vi "ChangeGrating.vi"(8 "error in (no error)":errorcluster, 10 "Grating":enum16{"Mirror", "1200 g/mm", "1800 g/mm"}(ring), 11 "HRS_Spectrometer in":refnum<class "HRS_Spectrometer.lvclass">) -> (0 "error out":errorcluster, 3 "HRS_Spectrometer out":refnum<class "HRS_Spectrometer.lvclass">)   [LabVIEW 2023, in "HRS_Spectrometer.lvlib" / "HRS_Spectrometer.lvclass"]
uses:
  HRS_Spectrometer.lvclass
  HRS_Spectrometer.lvclass/HRS_Spectrometer.ctl
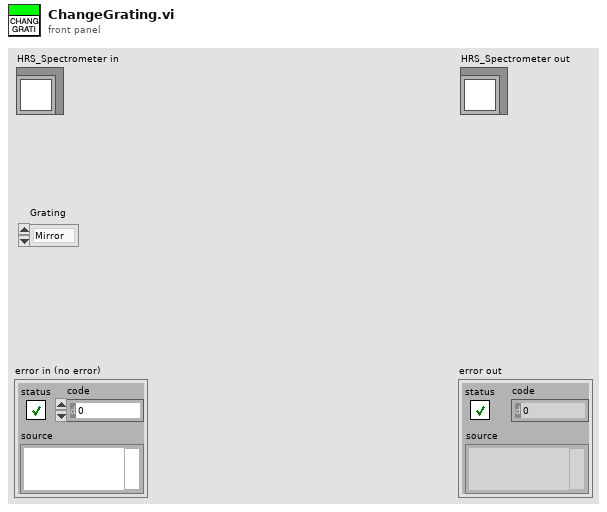
[diagram p1: front panel]
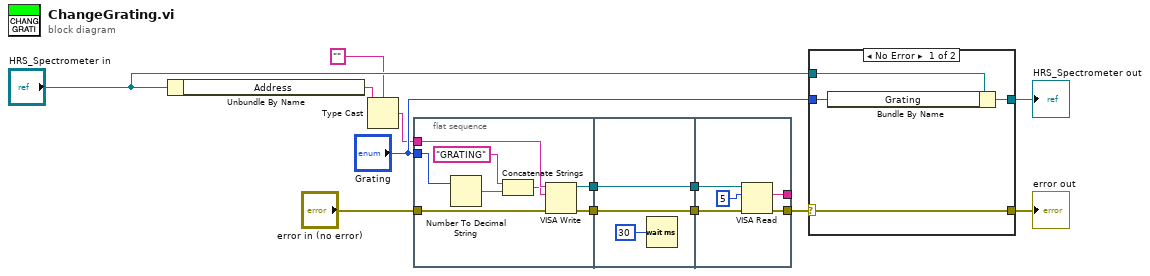
[diagram p0: block diagram]
diagram:
  n1 = Unbundle By Name("HRS_Spectrometer in") -> ("Address"=w3:string)
  n2 = Type Cast(type="", x=w3) -> (*(type *) &x=w1:string)
  n3 = flat-sequence {
    tunnel: [w21] -> w13
    tunnel: [w20] -> w12
    tunnel: "Grating" -> [w17]
    tunnel: w1 -> [w16]
    tunnel: "error in (no error)" -> [w15]
    tunnel: w13 -> [w24]
    tunnel: w12 -> [w23]
    tunnel: [w24] -> w11
    tunnel: [w23] -> w10
    tunnel: w11 -> [w28]
    tunnel: w10 -> [w29]
    tunnel: [w27] -> _
    tunnel: [w26] -> w9
    frame #0 {
      n4 = Number To Decimal String(number=w17) -> (decimal integer string=w18:string)  [unwired: 1 in]
      n5 = Concatenate Strings("GRATING" ("write buffer"), w18) -> (w14:string)
      n6 = VISA Write(VISA resource name=w16, write buffer=w14, error in (no error)=w15) -> (VISA resource name out=w21:refnum<visa-resource-name>, error out=w20:errorcluster)  [unwired: 1 out]
    }
    frame #1 {
      n7 = Wait (ms)(milliseconds to wait=u32 30) -> ()  [unwired: 1 out]
    }
    frame #2 {
      n8 = VISA Read(VISA resource name=w28, byte count=u32 5, error in (no error)=w29) -> (read buffer=w27:string, error out=w26:errorcluster)  [unwired: 2 out]
    }
  }
  n9 = case shown="No Error" w9 {
    selector: w9 -> [w30 w34]
    tunnel: "HRS_Spectrometer in" -> [w33 w35]
    tunnel: "Grating" -> [w32 _]
    tunnel: [w31 w35] -> w7
    tunnel: [w30 w34] -> w4
    frame No Error {
      n10 = Bundle By Name(cluster=w33, "Grating"=w32) -> (w31:refnum<class "HRS_Spectrometer.lvclass">)
    }
    frame Error {
    }
  }
  "error out" <- w4
  "HRS_Spectrometer out" <- w7
